vi "Periodic Tasks.vi"(8 "error in":errorcluster) -> ()   [LabVIEW 2019]
doc: "This VI runs in parallel to other robot code. It can contain as many user-defined periodic loops as you need. These can carry out PID or other sorts of timed response."
uses:
  Robot Global Data.vi
  <vilib>/Rock Robotics/WPI/Ultrasonic/WPI_SonarMB1010DigitalRefNum Registry Get.vi
  <vilib>/Rock Robotics/WPI/Ultrasonic/WPI_SonarMB1010DigitalGetRange.vi
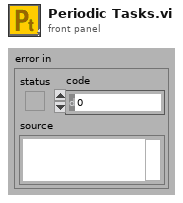
[diagram p1: front panel]
types:
  T1 = typedef "ADIS16448 Device Reference.ctl" = cluster{"DevStatus":errorcluster, "Hardware Config":T2, "Calibration Complete":refnum<notifier>, "Status FIFO":refnum<k33>, "Last Value Reference":refnum<data-value>, "Sychronous Process VI":T6, "Cmd FIFO":refnum<k33>, "Source":T7, "Data FIFO":refnum<k33>, "IMU Status LED Pin":T4, "Calibration Time":u32}
  T2 = typedef "ADIS16448 Hardware Configuration.ctl" = cluster{"SPI Clock Rate (Hz)":dbl, "IMU SPI Mode (3)":T3, "IMU Reset Pin":T4, "IMU SPI Bus":T5, "IMU Data Ready Pin":T4, "Stall Config":cluster{"Pow2BytesPerRead":u8, "StallTicks":u16, "CsToSclkTicks":u8}, "IMU Status LED Pin":T4}
  T3 = typedef "WPI_SPIMode.ctl" = enum16{"Mode 0 (Clk Idle Low,Sample on Leading)", "Mode 1 (Clk Idle Low,Sample on Trailing)", "Mode 2 (Clk Idle High,Sample on Leading)", "Mode 3 (Clk Idle High,Sample on Trailing)"}
  T4 = typedef "FPGA_DIOChannel.ctl" = enum8{"DIO 0", "DIO 1", "DIO 2", "DIO 3", "DIO 4", "DIO 5", "DIO 6", "DIO 7", "DIO 8", "DIO 9", "DIO MXP 0", "DIO MXP 1", "DIO MXP 2", "DIO MXP 3", "DIO MXP 4", "DIO MXP 5", "DIO MXP 6", "DIO MXP 7", "DIO MXP 8", "DIO MXP 9", "DIO MXP 10", "DIO MXP 11", "DIO MXP 12", "DIO MXP 13", "DIO MXP 14", "DIO MXP 15", "SPI Port CS1", "SPI Port CS2", "SPI Port CS3", "SPI Port MISO", "SPI Port MOSI", "Invalid"}
  T5 = typedef "spi_bus.ctl" = enum16{"SPI On-Board, CS0", "SPI On-Board, CS1", "SPI On-Board, CS2", "SPI On-Board, CS3", "SPI MXP", "Invalid"}
  T6 = typedef "ADIS16448 Process.ctl" = refnum<vi>
  T7 = typedef "FPGA_CounterEncoderSourceConvertionLVSourceType.ctl" = cluster{"DevStatus":errorcluster, "AnalogTriggerMode?":bool, "DigitalMode":cluster{"DIO Channel":T8}, "AnalogTriggerMode":cluster{"AnalogTriggerIndex":T9, "OutputType":T10}}
  T8 = typedef "FPGA_DIODigitalSourceChannel.ctl" = enum8{"DIO 0", "DIO 1", "DIO 2", "DIO 3", "DIO 4", "DIO 5", "DIO 6", "DIO 7", "DIO 8", "DIO 9", "DIO MXP 0", "DIO MXP 1", "DIO MXP 2", "DIO MXP 3", "DIO MXP 4", "DIO MXP 5", "DIO MXP 6", "DIO MXP 7", "DIO MXP 8", "DIO MXP 9", "DIO MXP 10", "DIO MXP 11", "DIO MXP 12", "DIO MXP 13", "DIO MXP 14", "DIO MXP 15", "SPI Port CS1", "SPI Port CS2", "SPI Port CS3", "SPI Port MISO", "SPI Port MOSI", "Disabled"}
  T9 = typedef "FPGA_AnalogTriggerIndex.ctl" = enum8{"Trig 0", "Trig 1", "Trig 2", "Trig 3", "Trig 4", "Trig 5", "Trig 6", "Trig 7", "Invalid"}
  T10 = typedef "FPGA_AnalogTriggerOutType.ctl" = enum16{"InWindow", "TriggerState", "Rising", "Falling"}
  T11 = typedef "WPI_JoystickDevRef.ctl" = cluster{"Device":T12}
  T12 = typedef "WPI_JoystickDeviceEnum.ctl" = enum16{"USB 0", "USB 1", "USB 2", "USB 3", "USB 4", "USB 5"}
  T13 = cluster{"JoystickDevRef":T11, "JoystickDevRef":T11, "ADIS16448DevRef Out":T1}
  T14 = typedef "WPI_SonarMB1010DigitalDeviceRef.ctl" = cluster{"CounterDevRef":T15, "Scaling factor (s/in)":dbl}
  T15 = typedef "WPI_CounterDevRef.ctl" = cluster{"DevStatus":errorcluster, "CntIndex":T16}
  T16 = typedef "FPGA_CounterCtrSystemIndex.ctl" = enum8{"Ctr 0", "Ctr 1", "Ctr 2", "Ctr 3", "Ctr 4", "Ctr 5", "Ctr 6", "Ctr 7", "Invalid"}
  T17 = typedef "ADIS16448 Data.ctl" = cluster{"XAngle":dbl, "YAngle":dbl, "ZAngle":dbl}
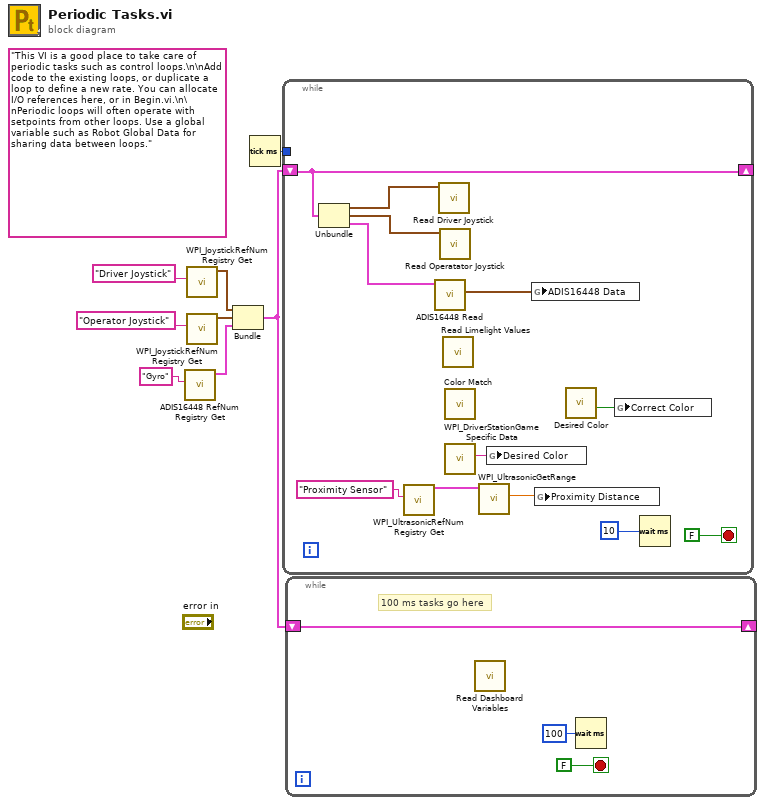
[diagram p0: block diagram]
diagram:
  (unwired) "This VI is a good place to take care of periodic tasks such as control loops.\n\nAdd code to the existing loops, or duplicate a loop to define a new rate. You can allocate I/O references here, or in Begin.vi.\n\nPeriodic loops will often operate with setpoints from other loops. Use a global variable such as Robot Global Data for sharing data between loops."
  n1 = call <vilib>:"ADIS16448 RefNum Registry Get.vi"("refnum name"="Gyro") -> ("ADIS16448DevRef Out"=w1:T1)  [unwired: 9 in, 1 out]
  n2 = call <vilib>:"WPI_JoystickRefNum Registry Get.vi"("refnum name"="Driver Joystick") -> ("JoystickDevRef"=w4:T11)  [unwired: 1 in, 9 out]
  n3 = call <vilib>:"WPI_JoystickRefNum Registry Get.vi"("refnum name"="Operator Joystick") -> ("JoystickDevRef"=w5:T11)  [unwired: 1 in, 9 out]
  n4 = Bundle("JoystickDevRef"=w4, "JoystickDevRef"=w5, "ADIS16448DevRef Out"=w1) -> (w3:T13)  [unwired: 1 in]
  n5 = Tick Count (ms)() -> (millisecond timer value=w7:u32)
  n6 = while {
    shift-right: [w18] -> _
    shift-left: w3 -> [w18]
    tunnel: w7 -> [_]
    stop <- FALSE stop-if-true
    n7 = Unbundle(w18) -> ("JoystickDevRef"=w17:T11, "JoystickDevRef"=w16:T11, "ADIS16448DevRef Out"=w15:T1)
    n8 = call-poly <vilib>:"WPI_UltrasonicRefNum Registry Get.vi"("refnum name"="Proximity Sensor") -> ("SonarMB1010DigitalDevRef"=w10:T14)  [unwired: 9 in, 1 out]
    n9 = call <vilib>:"ADIS16448 Read.vi"("ADIS16448DevRef"=w15) -> ("ADIS16448 Value"=w14:T17)  [unwired: 7 in, 3 out]
    n10 = call "Read Driver Joystick.vi"("Driver Joystick"=w17) -> ()  [unwired: 11 in]
    n11 = call "Read Operatator Joystick.vi"("Operator Joystick"=w16) -> ()  [unwired: 11 in]
    n12 = call "Read Limelight Values.vi"() -> ()  [unwired: 12 in]
    n13 = call "Color Match.vi"() -> ()  [unwired: 12 in]
    n14 = call <vilib>:"WPI_DriverStationGame Specific Data.vi"() -> ("Game Specific Data"=w13:string)  [unwired: 11 in]
    n15 = call-poly <vilib>:"WPI_UltrasonicGetRange.vi"("SonarMB1010DigitalDevRef"=w10) -> ("Distance"=w11:dbl)  [unwired: 8 in, 2 out]
    n16 = global write "Robot Global Data.vi" "Desired Color"(w13) -> ()
    n17 = global write "Robot Global Data.vi" "ADIS16448 Data"(w14) -> ()
    n18 = global write "Robot Global Data.vi" "Proximity Distance"(w11) -> ()
    n19 = call "Desired Color.vi"() -> ("Correct Color"=w12:bool)  [unwired: 10 in, 1 out]
    n20 = global write "Robot Global Data.vi" "Correct Color"(w12) -> ()
    n21 = Wait (ms)(milliseconds to wait=u32 10) -> ()  [unwired: 1 out]
  }
  n22 = while {
    shift-right: [w21] -> _
    shift-left: w3 -> [w21]
    stop <- FALSE stop-if-true
    # "100 ms tasks go here"
    n23 = call "Read Dashboard Variables.vi"() -> ()  [unwired: 12 in]
    n24 = Wait (ms)(milliseconds to wait=u32 100) -> ()  [unwired: 1 out]
  }
